vi "Machine_Data.vi"(8 "error in (no error)":errorcluster, 11 "Part?":bool) -> (0 "error out":errorcluster)   [LabVIEW 2020]
uses:
  Controls/Routing.ctl
  <menus>/Controls/Devaseelan Style/ONOFF Small.ctl
  <vilib>/addons/database/Connection.llb/Conn Execute.vi
  <vilib>/addons/database/NI_Database_API.lvlib
panel:
  out "Header":string
  in  "Save":bool
  in  "Exit":bool
  in  "Data":T1[](array[typedef])
  # "DB Table\nCode"
  # "Operation\nCode"
  # "Machine\nCode"
  # "Operation\nRequired"
  # "Pokayoke\nAllowed"
  # "S.No"
  # "Traceability"
  # "Engraving"
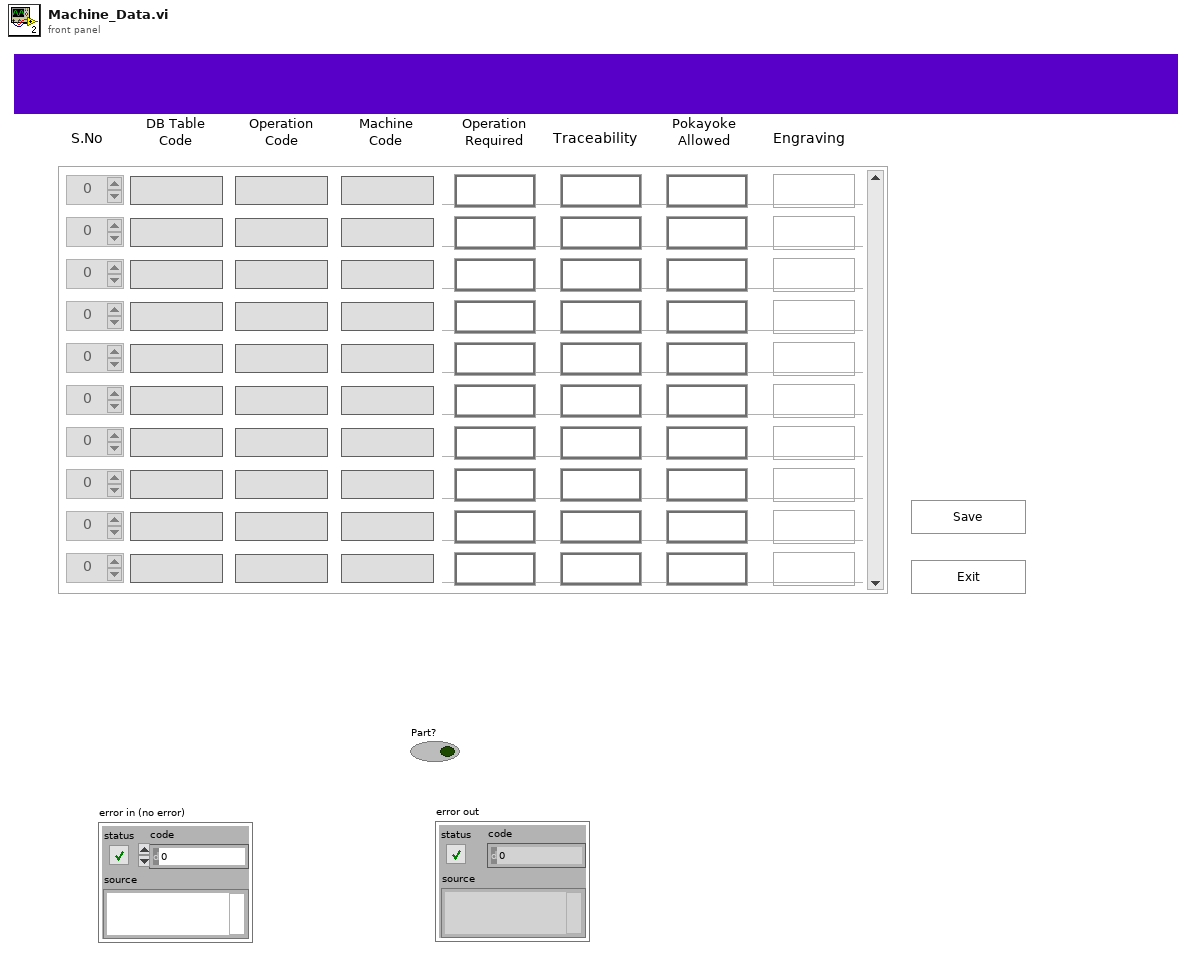
[diagram p1: front panel]
types:
  T1 = typedef "Routing.ctl" = cluster{"OperationSeqNo":i32, "Table Code":string, "OperationCode":string, "MachineCode":string, "OperationRequired":T2, "Traceability":T2, "POKA_YOKE_ALLOWED":T2, "Engraving":T2}
  T2 = typedef "ONOFF Small.ctl" = bool
  T3 = cluster{"Tag":string, "Checked":bool, "Enable":bool, "Name":string}[]
  T4 = typedef "TD SQL.ctl" = cluster{"MS SQL Connection":T5, "UDL File":path, "Time":string, "DCODE":string, "WIP+1":i64, "MC No?":i32, "POKAYOKE?":bool, "Expected Result":string, "Result [Status]":string, "Clock":dbl, "RFID":string, "WIP Queue":refnum<queue>, "TS Parameter":T6, "Data_Queue":refnum<queue>[], "RFID Serial No.":string}
  T5 = typedef "NI_Database_API.lvlib/Conn ObjectReference.ctl" = refnum<k1>
  T6 = typedef "TS_Parameter.ctl" = cluster{"ProfitCenterCode":string, "LineCode":string, "WorkOrderNumber":string, "Model":string, "Model_with_Prefix":string, "VendorCode":string, "SetParameterDateCode":string, "PokaYoke":i32, "Target":i32, "Live_DateCode":string, "CustomerPartNumber":string, "Hand":string, "sBarcode":bool, "FCA":i32, "Ent_Stamp":timestamp, "STS_CD":dbl}
  T7 = typedef "LVPoint32TypeDef.ctl" = cluster{"Horizontal":i32, "Vertical":i32}
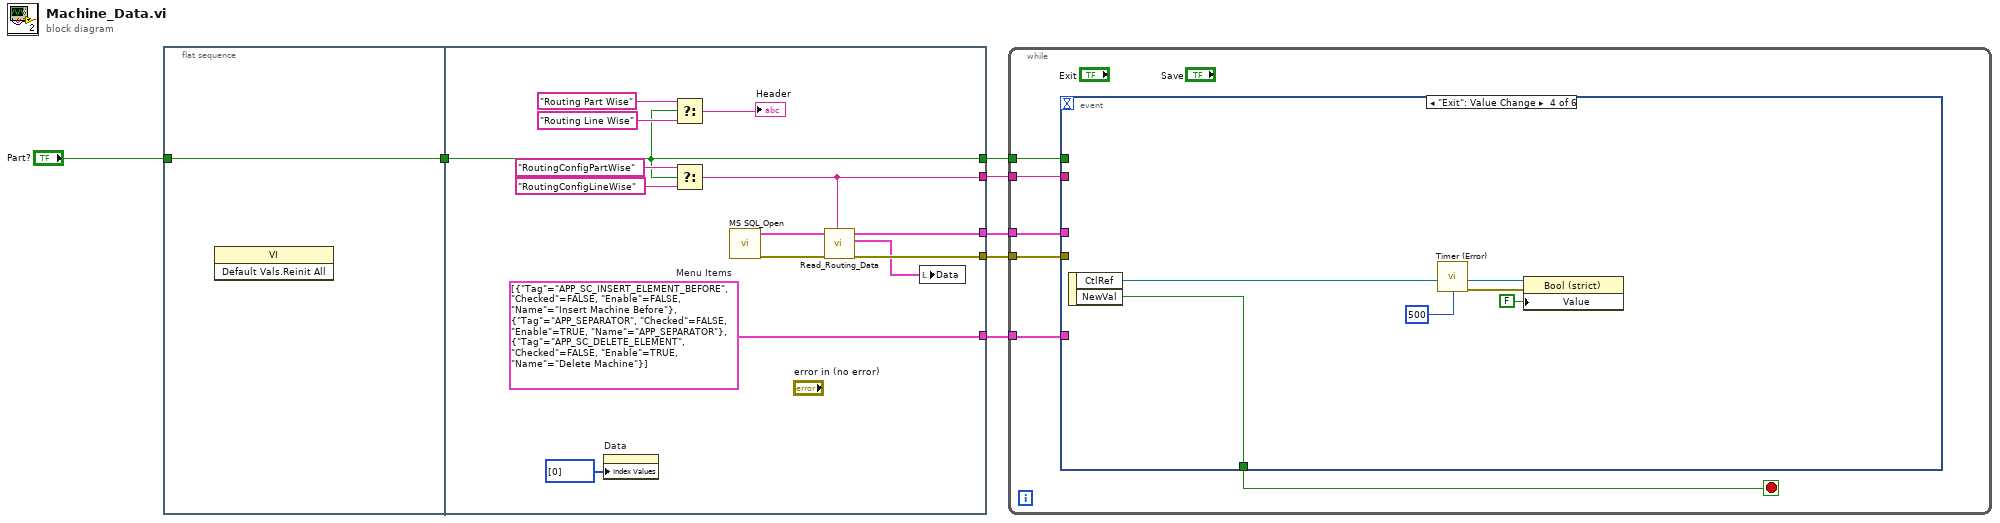
[diagram p0: block diagram]
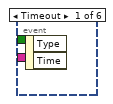
[diagram p2: hidden frame]
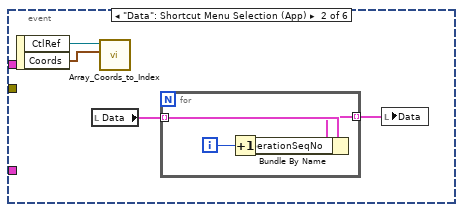
[diagram p3: hidden frame]
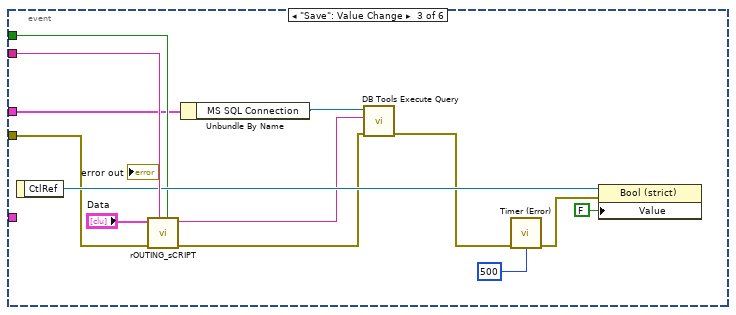
[diagram p4: hidden frame]
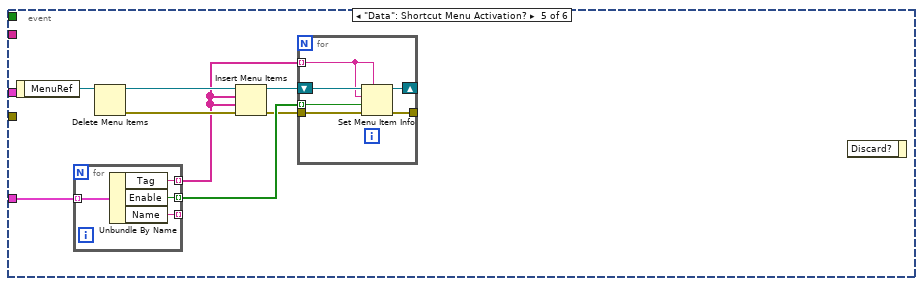
[diagram p5: hidden frame]
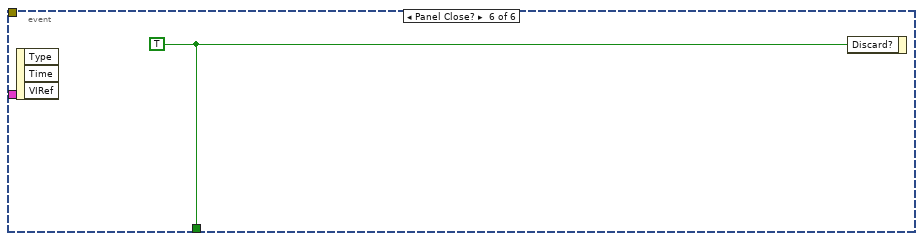
[diagram p6: hidden frame]
diagram:
  n1 = flat-sequence {
    tunnel: "Part?" -> [w8]
    tunnel: [w8] -> w1
    tunnel: [w20] -> w7
    tunnel: [w22] -> w6
    tunnel: [w18] -> w3
    tunnel: [w14] -> w5
    tunnel: [w11] -> w4
    tunnel: w1 -> [w11]
    frame #0 {
      n2 = invoke class="VI" method="Default Vals.Reinit All"() -> ()  [unwired: 3 in, 3 out]
    }
    frame #1 {
      w22 = T3 [{"Tag"="APP_SC_INSERT_ELEMENT_BEFORE", "Checked"=FALSE, "Enable"=FALSE, "Name"="Insert Machine Before"}, {"Tag"="APP_SEPARATOR", "Checked"=FALSE, "Enable"=TRUE, "Name"="APP_SEPARATOR"}, {"Tag"="APP_SC_DELETE_ELEMENT", "Checked"=FALSE, "Enable"=TRUE, "Name"="Delete Machine"}]  # Menu Items
      n3 = property on="Data" class="Arr (strict)"("Index Values"=u32[] [0]) -> ()  [unwired: 2 in, 2 out]
      n4 = Select(t="Routing Part Wise" ("table"), s=w11, f="Routing Line Wise" ("table")) -> (s? t:f=→"Header":string)
      n5 = Select(t="RoutingConfigPartWise" ("table"), s=w11, f="RoutingConfigLineWise" ("table")) -> (s? t:f=w14:string)
      n6 = call "MS SQL_Open.vi"() -> ("error out"=w21:errorcluster, "Ref Out"=w19:T4)  [unwired: 9 in, 1 out]
      n7 = call "Read_Routing_Data.vi"("table"=w14, "error in (no error)"=w21, "Ref In"=w19) -> ("error out"=w20:errorcluster, "Routing Data"=w17:T1[], "Ref Out"=w18:T4)  [unwired: 6 in]
      n8 = local write "Data"(w17) -> ()
    }
  }
  n9 = while {
    tunnel: w7 -> [w27]
    tunnel: w6 -> [w26]
    tunnel: w5 -> [w25]
    tunnel: w4 -> [w24]
    tunnel: w3 -> [w23]
    stop <- w28 stop-if-true
    n10 = event shown="[3] \"Exit\": Value Change" {
      selector: _ -> [_ _ _ _ _ _]
      dyn-events: _ -> [_ _ _ _ _ _]
      timeout: _ -> [_ _ _ _ _ _]
      tunnel: [_ _ _ w54 _ w73] -> w28
      tunnel: w27 -> [_ _ w39 _ _ _]
      tunnel: w26 -> [_ _ _ _ w61 _]
      tunnel: w25 -> [_ _ w49 _ _ _]
      tunnel: w24 -> [_ _ w43 _ _ _]
      tunnel: w23 -> [_ _ w42 _ _ _]
      event Timeout {
        n11 = event-data() -> ()  [unwired: 1 in, 2 out]
      }
      event "Data": Shortcut Menu Selection (App) {
        n12 = event-data() -> ("CtlRef"=w32:refnum<vi>, "Coords"=w31:T7)  [unwired: 1 in]
        n13 = local read "Data"() -> (w30:T1[])
        n14 = call "Array_Coords_to_Index.vi"("coords"=w31, "Array ref"=w32) -> ()  [unwired: 2 in, 4 out]
        n15 = for {
          tunnel: w30 -> [w36] mode=indexing
          tunnel: [w33] -> w29 mode=indexing
          i -> [w35]
          n16 = Increment(x=w35) -> (x+1=w34:i32)
          n17 = Bundle By Name(cluster=w36, "OperationSeqNo"=w34) -> (w33:T1)
        }
        n18 = local write "Data"(w29) -> ()
      }
      event "Save": Value Change {
        n19 = event-data() -> ("CtlRef"=w47:refnum<vi>)  [unwired: 1 in]
        n20 = call "rOUTING_sCRIPT.vi"("Part?"=w43, "Table"=w49, "error in (no error)"=w39, "Data"="Data") -> ("error out"=w37:errorcluster, "spreadsheet string"=w40:string)  [unwired: 6 in]
        n21 = Unbundle By Name(w42) -> ("MS SQL Connection"=w41:T5)
        n22 = call-poly <vilib>:"DB Tools Execute Query.vi"("error in (no error)"=w37, "SQL query"=w40, "connection reference"=w41) -> ("error out"=w38:errorcluster)  [unwired: 5 in, 1 out]
        n23 = call <userlib>:"Timer (Error).vi"("error in (no error)"=w38, "milliseconds to wait"=u32 500) -> ("error out"=w44:errorcluster)  [unwired: 13 in]
        n24 = property class="Bool (strict)"(reference=w47, error in=w44, "Value"=FALSE) -> ()  [unwired: 2 out]
      }
      event "Exit": Value Change {
        n25 = event-data() -> ("CtlRef"=w50:refnum<vi>, "NewVal"=w54:bool)  [unwired: 1 in]
        n26 = call <userlib>:"Timer (Error).vi"("milliseconds to wait"=u32 500) -> ("error out"=w51:errorcluster)  [unwired: 14 in]
        n27 = property class="Bool (strict)"(reference=w50, error in=w51, "Value"=FALSE) -> ()  [unwired: 2 out]
      }
      event "Data": Shortcut Menu Activation? {
        n28 = event-data() -> ("MenuRef"=w62:refnum<k9>)  [unwired: 1 in]
        n29 = for {
          tunnel: w61 -> [w72] mode=indexing
          tunnel: [w71] -> w55 mode=indexing
          tunnel: [w70] -> w58 mode=indexing
          tunnel: [w69] -> _ mode=indexing
          n30 = Unbundle By Name(w72) -> ("Tag"=w71:string, "Enable"=w70:bool, "Name"=w69:string)
        }
        n31 = Delete Menu Items(9:w62) -> (0:w57:errorcluster, 3:w60:refnum<k9>)  [unwired: 3 in]
        n32 = Insert Menu Items(6:w57, 7:w55, 8:w55, 9:w60) -> (0:w56:errorcluster, 3:w59:refnum<k9>)  [unwired: 2 in, 1 out]
        n33 = for {
          tunnel: [w67] -> _
          tunnel: w55 -> [w63] mode=indexing
          tunnel: w58 -> [w66] mode=indexing
          shift-right: [w65] -> _
          shift-left: w59 -> [w68]
          tunnel: w56 -> [w64]
          n34 = Set Menu Item Info(7:w63, 8:w64, 9:w66, 10:w63, 11:w68) -> (0:w67:errorcluster, 3:w65:refnum<k9>)  [unwired: 2 in]
        }
        n35 = event-data() -> ()  [unwired: 2 in, 1 out]
      }
      event Panel Close? {
        w73 = TRUE ("Discard?")
        n36 = event-data() -> ()  [unwired: 1 in, 3 out]
        n37 = event-data("Discard?"=w73) -> ()  [unwired: 1 in, 1 out]
      }
    }
  }
